vi "Configure Hardware.vi"(8 "error in (no error)":errorcluster, 11 "Hardware Resources In":T1={"Piezo Serial Number"=41848555, "MG17Piezo"=refnum, "Setpoint (um)"=0.0}) -> (0 "error out":errorcluster, 3 "Hardware Resources Out":T1={"Piezo Serial Number"=41848555, "MG17Piezo"=refnum, "Setpoint (um)"=0.0})   [LabVIEW 2013, in "Piezo.lvlib"]
uses:
  Piezo.lvlib
  Hardware Configuration.ctl
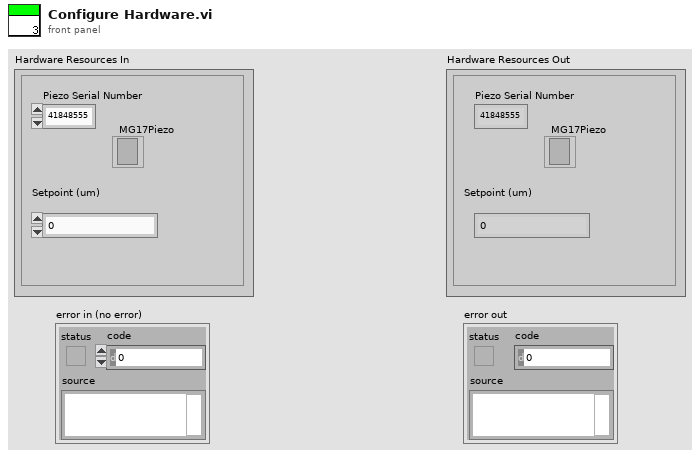
[diagram p1: front panel]
types:
  T1 = typedef "Piezo.lvlib/Hardware Configuration.ctl" = cluster{"Piezo Serial Number":i32, "MG17Piezo":refnum<k7>, "Setpoint (um)":sgl}
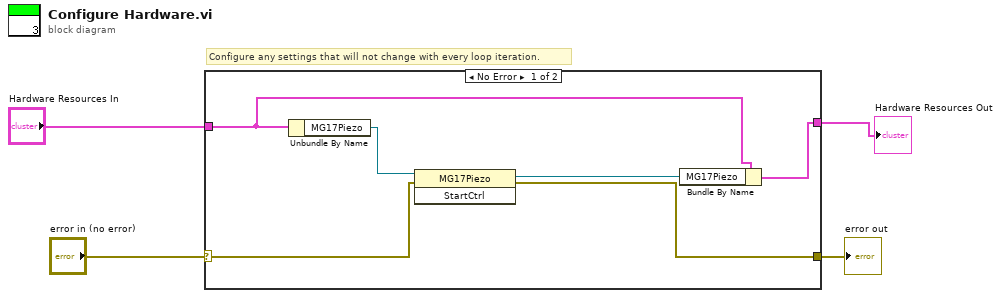
[diagram p0: block diagram]
diagram:
  # "Configure any settings that will not change with every loop iteration."
  n1 = case shown="No Error" "error in (no error)" {
    selector: "error in (no error)" -> [w5 w12]
    tunnel: [w6 w12] -> w3
    tunnel: [w8 w11] -> w1
    tunnel: "Hardware Resources In" -> [w9 w11]
    frame No Error {
      n2 = Unbundle By Name(w9) -> ("MG17Piezo"=w10:refnum<k7>)
      n3 = invoke class="MG17Piezo" method="StartCtrl"(reference=w10, error in=w5) -> (reference out=w7:refnum<k7>, error out=w6:errorcluster)  [unwired: 1 in, 1 out]
      n4 = Bundle By Name(cluster=w9, "MG17Piezo"=w7) -> (w8:T1)
    }
    frame Error {
    }
  }
  "error out" <- w3
  "Hardware Resources Out" <- w1
